vi "arduinoCloseComPort.vi"(8 "Error In":errorcluster, 11 "VISA resource":refnum<visa-resource-name>) -> (0 "error out":errorcluster)   [LabVIEW 2019]
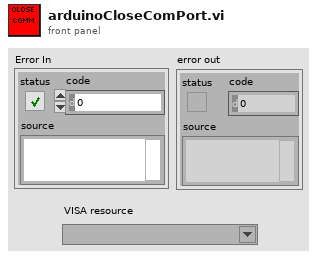
[diagram p1: front panel]
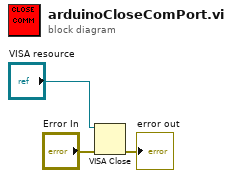
[diagram p0: block diagram]
diagram:
  n1 = VISA Close(VISA resource name="VISA resource", error in (no error)="Error In") -> (error out=→"error out":errorcluster)
